vi "Folder search from Path.vi"(8 "error in (no error)":errorcluster, 11 "path":path) -> (0 "error out":errorcluster, 3 "Folder Path":string)   [LabVIEW 2015, in "Data Saving.lvlib"]
uses:
  <vilib>/regexp/Match Regular Expression.xnode
  Generic Instrument/Data Saving/TDMS Saver/Data Saving.lvlib
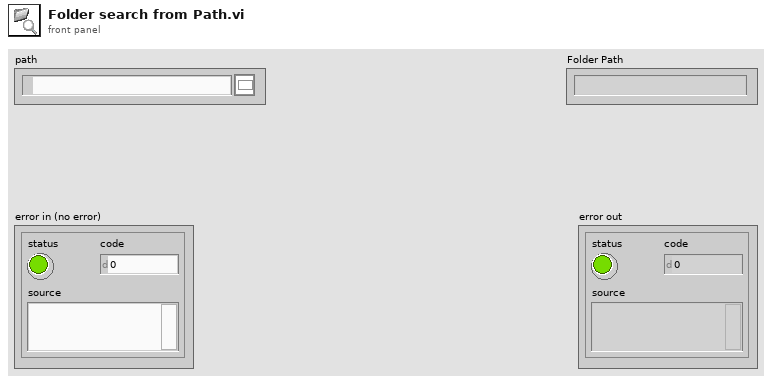
[diagram p1: front panel]
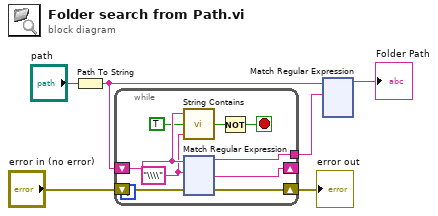
[diagram p0: block diagram]
diagram:
  n1 = Path To String(path="path") -> (string=w4:string)
  n2 = while {
    shift-right: [w12] -> _
    shift-left: w4 -> [w15]
    shift-right: [w10] -> w3
    shift-left: "error in (no error)" -> [w9]
    tunnel: [w8] -> w5
    stop <- w7 stop-if-true
    w14 = "\\\\" ("regular expression")
    n3 = call "String Contains.vi"("Regular expression"=w14, "Case Sensitive?"=TRUE, "Input String"=w15) -> ("Boolean"=w13:bool)  [unwired: 2 in]
    n4 = xnode "Match Regular Expression"("input string"=w15, "regular expression"=w14, "error in"=w9) -> ("before match"=w8:string, "after match"=w12:string, "error out"=w10:errorcluster)  [unwired: 3 in, 2 out]
    n5 = Not(x=w13) -> (.not. x?=w7:bool)
  }
  "error out" <- w3
  n6 = xnode "Match Regular Expression"("input string"=w4, "regular expression"=w5) -> ("before match"=→"Folder Path":string)  [unwired: 4 in, 4 out]
